vi "VolltagePeltierResonanceCurve.vi"(5 "#Measurements each Frequency":i32=200, 6 "Step":dbl=200.0 format="%.2f", 8 "error in":errorcluster, 9 "Stop":dbl=200.0 format="%.2f", 10 "Start":dbl=200.0 format="%.2f", 11 "Voltage":dbl=200.0 format="%.2f") -> (0 "error out":errorcluster)   [LabVIEW 2010]
panel:
  in  "Wait":dbl=200.0 format="%.2f"
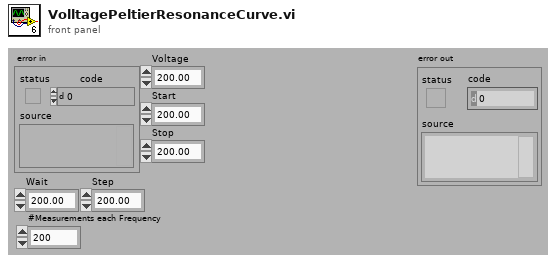
[diagram p1: front panel]
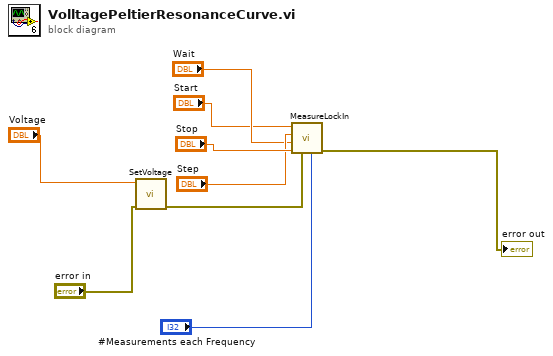
[diagram p0: block diagram]
diagram:
  n1 = call "SetVoltage.vi"("error in"="error in", "Voltage"="Voltage") -> ("error out"=w2:errorcluster)  [unwired: 9 in]
  n2 = call "MeasureLockIn.vi"("#Measurements each Frequency"="#Measurements each Frequency", "error in"=w2, "Stop"="Stop", "Wait (ms)"="Wait", "Step"="Step", "Start"="Start") -> ("error out"=→"error out":errorcluster)  [unwired: 5 in]
